vi "initializer_run.vi"(0 "Digital in":refnum<vi>, 1 "Bool Refnum":refnum<vi>, 2 "Simulation File":refnum<vi>, 3 "Run":refnum<vi>, 4 "Load Vali File":refnum<vi>, 5 "Validate":refnum<vi>, 6 "Dataflow Out":refnum<vi>, 8 "Cancel Button":refnum<vi>, 9 "Save Specs":refnum<vi>, 10 "reference 3":refnum<vi>, 11 "Refresh Button":refnum<vi>, 12 "Starttime":refnum<vi>, 13 "Load Simulation File":refnum<vi>, 14 "reference 2":refnum<vi>, 15 "Load Spec File":refnum<vi>, 16 "reference":refnum<vi>) -> (18 "Checkbox":bool)   [LabVIEW 2019]
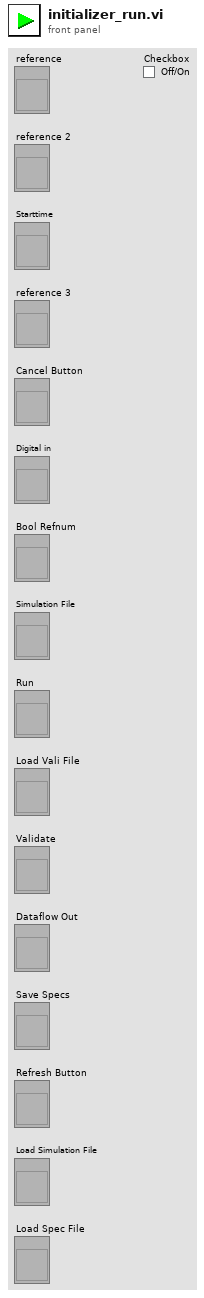
[diagram p1: front panel]
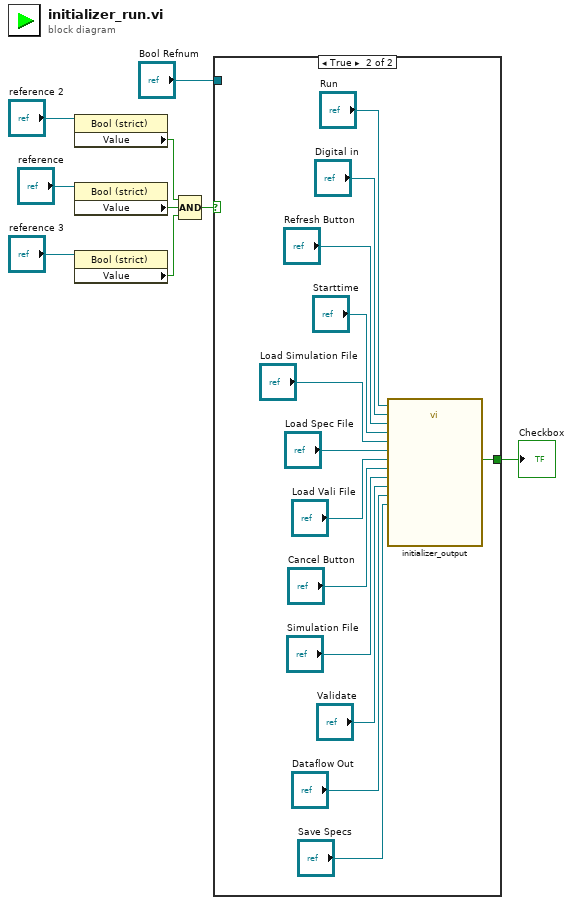
[diagram p0: block diagram]
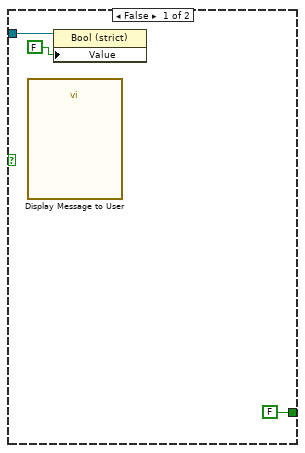
[diagram p2: hidden frame]
diagram:
  n1 = property class="Bool (strict)"(reference="reference 2") -> ("Value"=w5:bool)  [unwired: 1 in, 2 out]
  n2 = property class="Bool (strict)"(reference="reference") -> ("Value"=w6:bool)  [unwired: 1 in, 2 out]
  n3 = property class="Bool (strict)"(reference="reference 3") -> ("Value"=w7:bool)  [unwired: 1 in, 2 out]
  n4 = Compound Arithmetic op=AND(w5, w6, w7) -> (w8:bool)
  n5 = case shown="True" w8 {
    tunnel: [FALSE w25] -> w9
    tunnel: "Bool Refnum" -> [w10 _]
    frame False {
      n6 = call "Display Message to User"() -> ()  [unwired: 10 in, 2 out]
      n7 = property on="Property Node" class="Bool (strict)"(reference=w10, "Value"=FALSE ("Run")) -> ()  [unwired: 1 in, 2 out]
    }
    frame True {
      n8 = call "initializer_output.vi"("Boolean in"="Run", "reference 3"="Digital in", "Bool Refnum 4"="Refresh Button", "reference 2"="Starttime", "Bool Refnum 5"="Load Simulation File", "Bool Refnum 3"="Save Specs", "Bool Refnum 6"="Load Spec File", "reference 4"="Dataflow Out", "Bool Refnum 7"="Load Vali File", "Bool Refnum in"="Validate", "Bool Refnum 8"="Cancel Button", "reference"="Simulation File") -> ("Checkbox"=w25:bool)  [unwired: 7 in]
    }
  }
  "Checkbox" <- w9
